vi "Unsubscribe Wrapper.vi"(8 "error in (no error)":errorcluster, 11 "Reader Handle":i64) -> (0 "error out":errorcluster)   [LabVIEW 2021, in "Zenoh.lvclass"]
uses:
  <vilib>/CIF Foundation/CIF Utilities/Errors/Append Error Location.vi
  Zenoh.lvclass
  Zenoh.lvclass/Zenoh.ctl
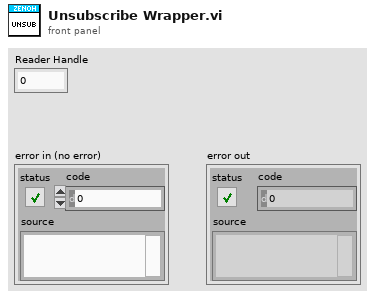
[diagram p1: front panel]
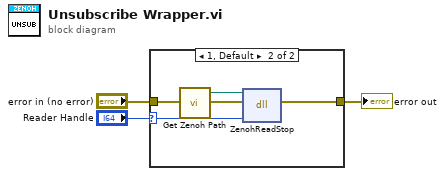
[diagram p0: block diagram]
diagram:
  n1 = case shown="1, Default" "Reader Handle" {
    selector: "Reader Handle" -> [_ w5]
    tunnel: "error in (no error)" -> [w4 w7]
    tunnel: [w4 w6] -> w2
    frame 0 {
    }
    frame 1, Default {
      n2 = call "Get Zenoh Path.vi"() -> ("Library Path"=w8:path)  [unwired: 4 in]
      n3 = dll-call lib="D:/dev/zenoh/wrapper/zenoh_wrapper_reader.dll" fn="ZenohReadStop"(path in=w8, error in=w7, "readerHandle"=w5) -> (error out=w6:errorcluster)  [unwired: 3 in, 1 out]
    }
  }
  "error out" <- w2
